vi "To Initialize Session Behavior.vi"(11 "initialize and close session behavior":T2) -> (3 "initialize session behavior":T1)   [LabVIEW 2020, in "MeasurementLink Instrument.lvlib" / "IInstrument.lvclass"]
uses:
  IInstrument.lvclass
  Initialize Session Behavior.ctl
  Initialize and Close Session Behavior.ctl
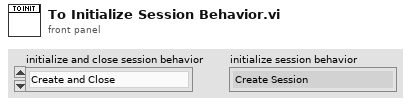
[diagram p1: front panel]
types:
  T1 = typedef "MeasurementLink Instrument.lvlib/IInstrument.lvclass/Initialize Session Behavior.ctl" = enum16{"Create Session", "Attach Session"}
  T2 = typedef "MeasurementLink Instrument.lvlib/IInstrument.lvclass/Initialize and Close Session Behavior.ctl" = enum16{"Create and Close", "Attach and Detach", "Create and Detach", "Attach and Close"}
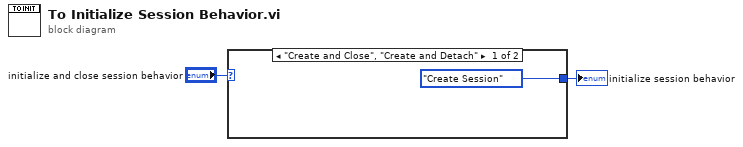
[diagram p0: block diagram]
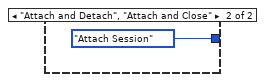
[diagram p2: hidden frame]
diagram:
  n1 = case shown="\"Create and Close\", \"Create and Detach\"" "initialize and close session behavior" {
    tunnel: [Initialize_Session_Behavior."Create Session" ("initialize session behavior 2") Initialize_Session_Behavior."Attach Session" ("initialize session behavior 2")] -> w1
    frame "Create and Close", "Create and Detach" {
    }
    frame "Attach and Detach", "Attach and Close" {
    }
  }
  "initialize session behavior" <- w1
